vi "write Port.vi"(9 "length":i32, 10 "packet":string, 11 "port_num":i32) -> (2 "packet out":string, 3 "function return":i32)   [LabVIEW 2015, in "dxl_x86_c.lvlib"]
doc: "WINDECLSPEC int writePort (int port_num, uint8_t *packet, int length);"
uses:
  dxl_x86_c.lvlib
  dxl_x86_c.dll
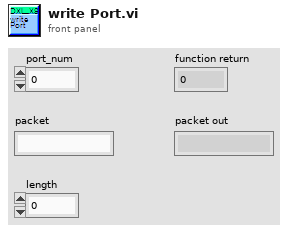
[diagram p1: front panel]
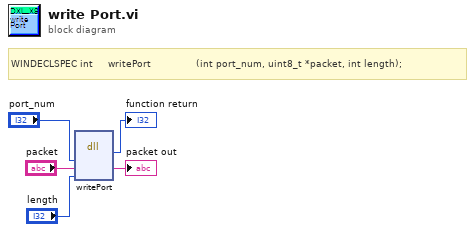
[diagram p0: block diagram]
diagram:
  # "WINDECLSPEC int     writePort               (int port_num, uint8_t *packet, int length);"
  n1 = dll-call lib="C:/Users/Platform/Desktop/LabVIEW/dxl_x86_c.lvlib/dxl_x86_c.*" fn="writePort"("port_num"="port_num", "packet"="packet", "length"="length") -> (→"function return":i32, "packet"=→"packet out":string)  [unwired: 5 in, 2 out]
